vi "Script CSV.vi"(8 "error in (no error)":errorcluster, 10 "dma block":T1(array[cluster]), 11 "path":path) -> (0 "error out":errorcluster)   [LabVIEW 2017]
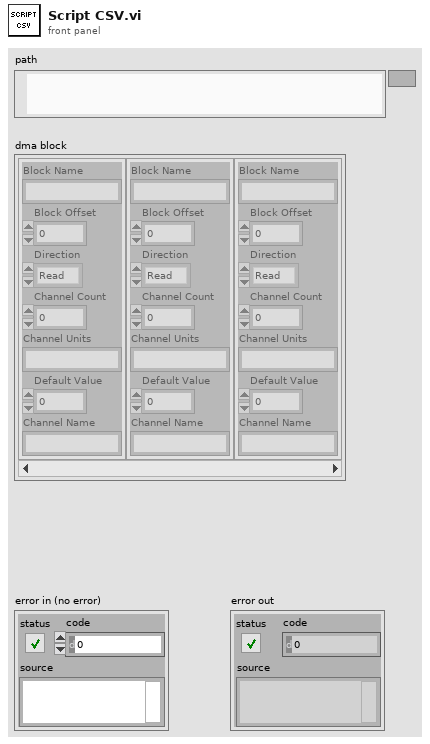
[diagram p1: front panel]
types:
  T1 = cluster{"Block Name":string, "Block Offset":u32, "Direction":enum16{"Read", "Write"}, "Channel Count":u32, "Channel Units":string, "Default Value":dbl, "Channel Name":string}[]
  T2 = cluster{"Channel Name":string, "Channel Units":string, "Default Value":dbl}
  T3 = cluster{"Block Name":string, "Block Offset":u32, "Direction":enum16{"Read", "Write"}, "Channels":cluster{"Channel Name":string, "Channel Units":string, "Default Value":dbl}[]}
  T4 = cluster{"Channel Name":string, "Channel Units":string, "Default Value":dbl}[]
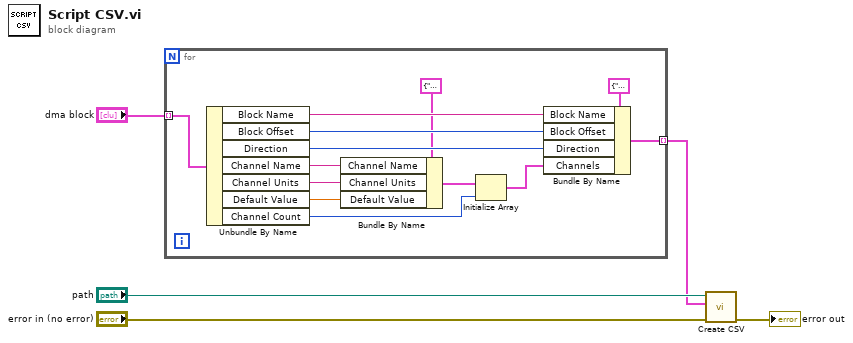
[diagram p0: block diagram]
diagram:
  n1 = for {
    tunnel: "dma block" -> [w18] mode=indexing
    tunnel: [w15] -> w1 mode=indexing
    n2 = Unbundle By Name(w18) -> ("Block Name"=w16:string, "Block Offset"=w14:u32, "Direction"=w13:enum16{"Read", "Write"}, "Channel Name"=w9:string, "Channel Units"=w10:string, "Default Value"=w11:dbl, "Channel Count"=w6:u32)
    n3 = Bundle By Name(cluster=T2 {"Channel Name"="", "Channel Units"="", "Default Value"=0.0} ("Channels"), "Channel Name"=w9, "Channel Units"=w10, "Default Value"=w11) -> (w8:T2)
    n4 = Initialize Array(w8, w6) -> (w7:T4)
    n5 = Bundle By Name(cluster=T3 {"Block Name"="", "Block Offset"=0, "Direction"=enum."Read", "Channels"=[{"Channel Name"="Channel", "Channel Units"="V", "Default Value"=0.0}]} ("dma blocks"), "Block Name"=w16, "Block Offset"=w14, "Direction"=w13, "Channels"=w7) -> (w15:T3)
  }
  n6 = call "Create CSV.vi"("error in (no error)"="error in (no error)", "dma blocks"=w1, "path"="path") -> ("error out"=→"error out":errorcluster)  [unwired: 8 in]
